vi "De-NaN Values.vi"(10 "Last Valid":dbl, 11 "Input":dbl) -> (3 "De-NaN":dbl)   [LabVIEW 2017]
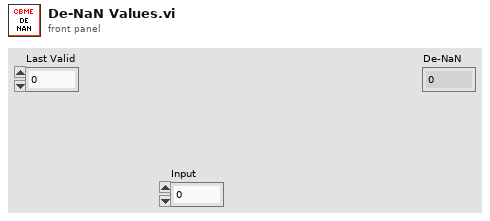
[diagram p1: front panel]
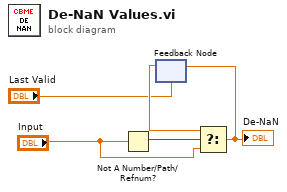
[diagram p0: block diagram]
diagram:
  n1 = Not A Number/Path/Refnum?(number/path/refnum="Input") -> (NaN/Path/Refnum?=w4:bool)
  n2 = feedback #1("Last Valid") -> (w2:dbl)
  n3 = Select(t=w2, s=w4, f="Input") -> (s? t:f=w3:dbl)
  "De-NaN" <- w3
  n4 = feedback-in #1(w3) -> ()
